vi "dataCorrector.vi"(0 "reference in":refnum<class "PartsTracking Controller.lvclass">, 5 "error in (no error)":errorcluster) -> (14 "reference out":refnum<class "PartsTracking Controller.lvclass">, 19 "error out":errorcluster)   [LabVIEW 2014, in "PartsTracking Controller.lvclass"]
uses:
  PartsTracking Controller.lvclass
  APP/excelFile_class/fileType.ctl
  APP/excelFile_class/excelFile.lvclass
  File Controller_llb/File Controller.lvclass
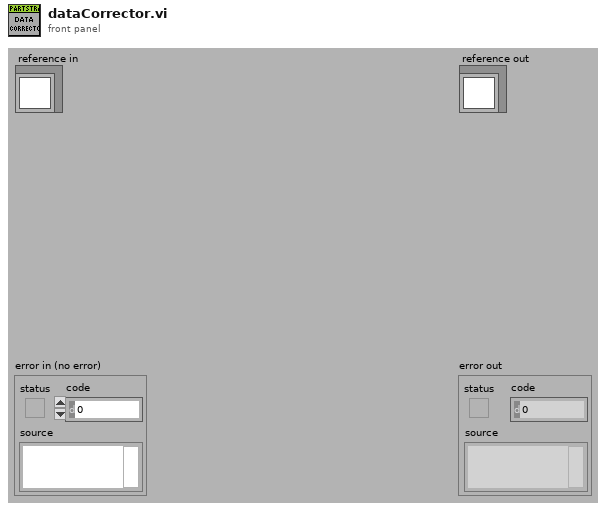
[diagram p1: front panel]
types:
  T1 = typedef "excelFile.lvclass/fileType.ctl" = enum16{"devices", "items", "partsTracking"}
  T2 = typedef "PartsTracking Controller.lvclass/ObjectAttributesRef.ctl" = refnum<data-value>
  T3 = typedef "PartsTracking Controller.lvclass/ObjectAttributes.ctl" = cluster{"MyAttribute":dbl, "file_controller_ref":refnum<class "File Controller.lvclass">, "data":string[][], "partsTracking_ref":refnum<class "partsTracking.lvclass">, "project_panels_ref":refnum<class "Project Panels.lvclass">}
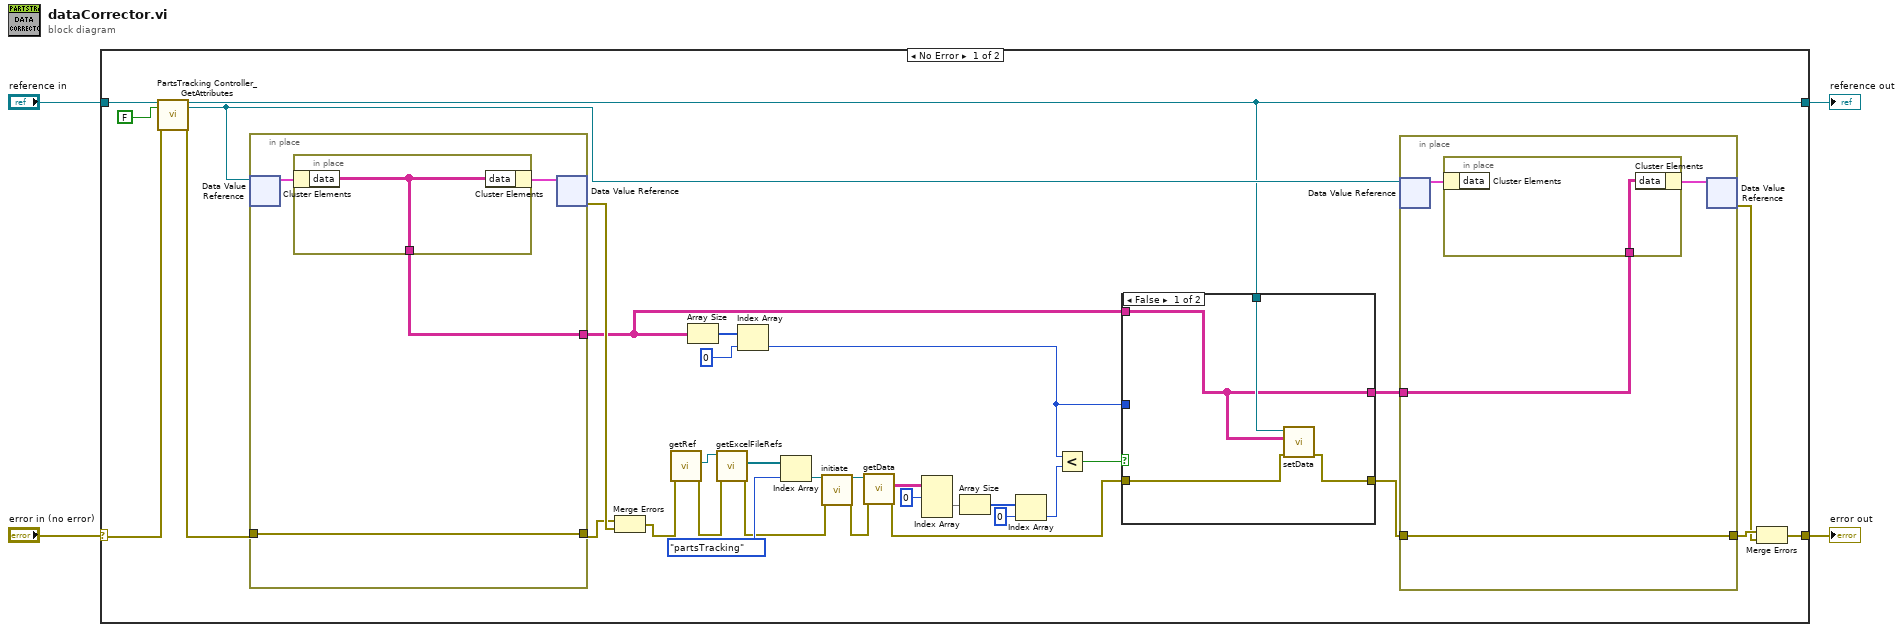
[diagram p0: block diagram]
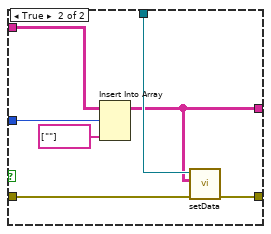
[diagram p2: hidden frame]
diagram:
  n1 = case shown="No Error" "error in (no error)" {
    selector: "error in (no error)" -> [w34 w61]
    tunnel: [w13 w61] -> w3
    tunnel: [w7 w60] -> w1
    tunnel: "reference in" -> [w36 w60]
    frame No Error {
      n2 = call "PartsTracking Controller_GetAttributes.vi"("reference in"=w36, "return data? (T)"=FALSE, "error in (no error)"=w34) -> ("reference out"=w7:refnum<class "PartsTracking Controller.lvclass">, "attributes ref"=w12:T2, "error out"=w33:errorcluster)  [unwired: 13 in, 1 out]
      n3 = in-place {
        in-place-border: w33 -> [w56]
        in-place-border: [w56] -> w37
        in-place-border: [w55] -> w10
        n4 = in-place-dvr #1(w12) -> (w57:T3)  [unwired: 1 out]
        n5 = in-place {
          in-place-border: [w59] -> w55
          n6 = in-place-cluster #2(w57) -> ("data"=w59:string[][])
          n7 = in-place-cluster #2("data"=w59) -> (w58:T3)
        }
        n8 = in-place-dvr #1(w58) -> (w38:errorcluster)  [unwired: 1 out]
      }
      n9 = Merge Errors(w37, w38) -> (w27:errorcluster)
      n10 = call "getRef.vi"("error in (no error)"=w27) -> ("error out"=w32:errorcluster, "File Controller_ref"=w25:refnum<class "File Controller.lvclass">)  [unwired: 9 in]
      n11 = Array Size(array=w10) -> (size(s)=w20:i32[])
      n12 = call "getExcelFileRefs.vi"("error in (no error)"=w32, "reference in"=w25) -> ("error out"=w22:errorcluster, "excelFile_refs"=w31:refnum<class "excelFile.lvclass">[])  [unwired: 7 in, 1 out]
      n13 = Index Array(array=w20, index=0) -> (element=w9:i32)
      n14 = Index Array(array=w31, index=fileType."partsTracking" ("fileType")) -> (element=w24:refnum<class "excelFile.lvclass">)
      n15 = call-dynamic "initiate.vi"("reference in"=w24, "error in (no error)"=w22) -> ("reference out"=w23:refnum<class "excelFile.lvclass">, "error out"=w21:errorcluster)  [unwired: 16 in]
      n16 = call "getData.vi"("error in (no error)"=w21, "reference in"=w23) -> ("error out"=w6:errorcluster, "data"=w30:string[][][])  [unwired: 7 in, 1 out]
      n17 = Index Array(array=w30, index (dim 0)=0 ("index (page)")) -> (element=w26:string[][])  [unwired: 2 in]
      n18 = Array Size(array=w26) -> (size(s)=w19:i32[])
      n19 = Index Array(array=w19, index=0) -> (element=w16:i32)
      n20 = Less?(x=w9, y=w16) -> (x < y?=w11:bool)
      n21 = case shown="False" w11 {
        tunnel: w10 -> [w41 w49]
        tunnel: w9 -> [_ w48]
        tunnel: [w41 w43] -> w8
        tunnel: w6 -> [w40 w46]
        tunnel: w7 -> [w42 w45]
        tunnel: [w39 w44] -> w5
        frame False {
          n22 = call "setData.vi"("error in (no error)"=w40, "Data"=w41, "reference in"=w42) -> ("error out"=w39:errorcluster)  [unwired: 7 in, 1 out]
        }
        frame True {
          n23 = Insert Into Array(array=w49, index (row)=w48, new element=string[] [""] ("new element/subarray")) -> (w43:string[][])  [unwired: 1 in]
          n24 = call "setData.vi"("error in (no error)"=w46, "Data"=w43, "reference in"=w45) -> ("error out"=w44:errorcluster)  [unwired: 7 in, 1 out]
        }
      }
      n25 = in-place {
        in-place-border: w5 -> [w51]
        in-place-border: [w51] -> w15
        in-place-border: w8 -> [w50]
        n26 = in-place-dvr #3(w12) -> (w52:T3)  [unwired: 1 out]
        n27 = in-place {
          in-place-border: w50 -> [w54]
          n28 = in-place-cluster #4(w52) -> ()  [unwired: 1 out]
          n29 = in-place-cluster #4("data"=w54) -> (w53:T3)
        }
        n30 = in-place-dvr #3(w53) -> (w14:errorcluster)  [unwired: 1 out]
      }
      n31 = Merge Errors(w15, w14) -> (w13:errorcluster)
    }
    frame Error {
    }
  }
  "error out" <- w3
  "reference out" <- w1
